vi "DMM_Global.vi"() -> ()   [LabVIEW 2018, in "DMM Virtual.lvclass"]
uses:
  DMM Virtual.lvclass
panel:
  in  "DMM_Refs":refnum<class "DMM Virtual.lvclass">[](array[class])
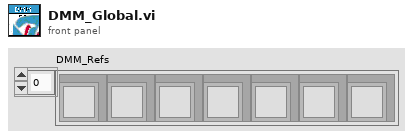
[diagram p1: front panel]
diagram:
